vi "Read_Spectro_Variant.vi"(8 "error in (no error)":errorcluster, 9 "Variant":variant, 10 "SpectroCluster":T1) -> (0 "error out":errorcluster, 2 "SpectroCluster":T1)   [LabVIEW 2023, in "Spectrometer Library.lvlib" / "SpectrometerUI.lvlib"]
uses:
  SpectrometerUI.lvlib
  typedefs/SpectroData.ctl
  <userlib>/_OpenG.lib/lvdata/lvdata.llb/openg_variant.lvlib
  typedefs/typedefs.lvlib
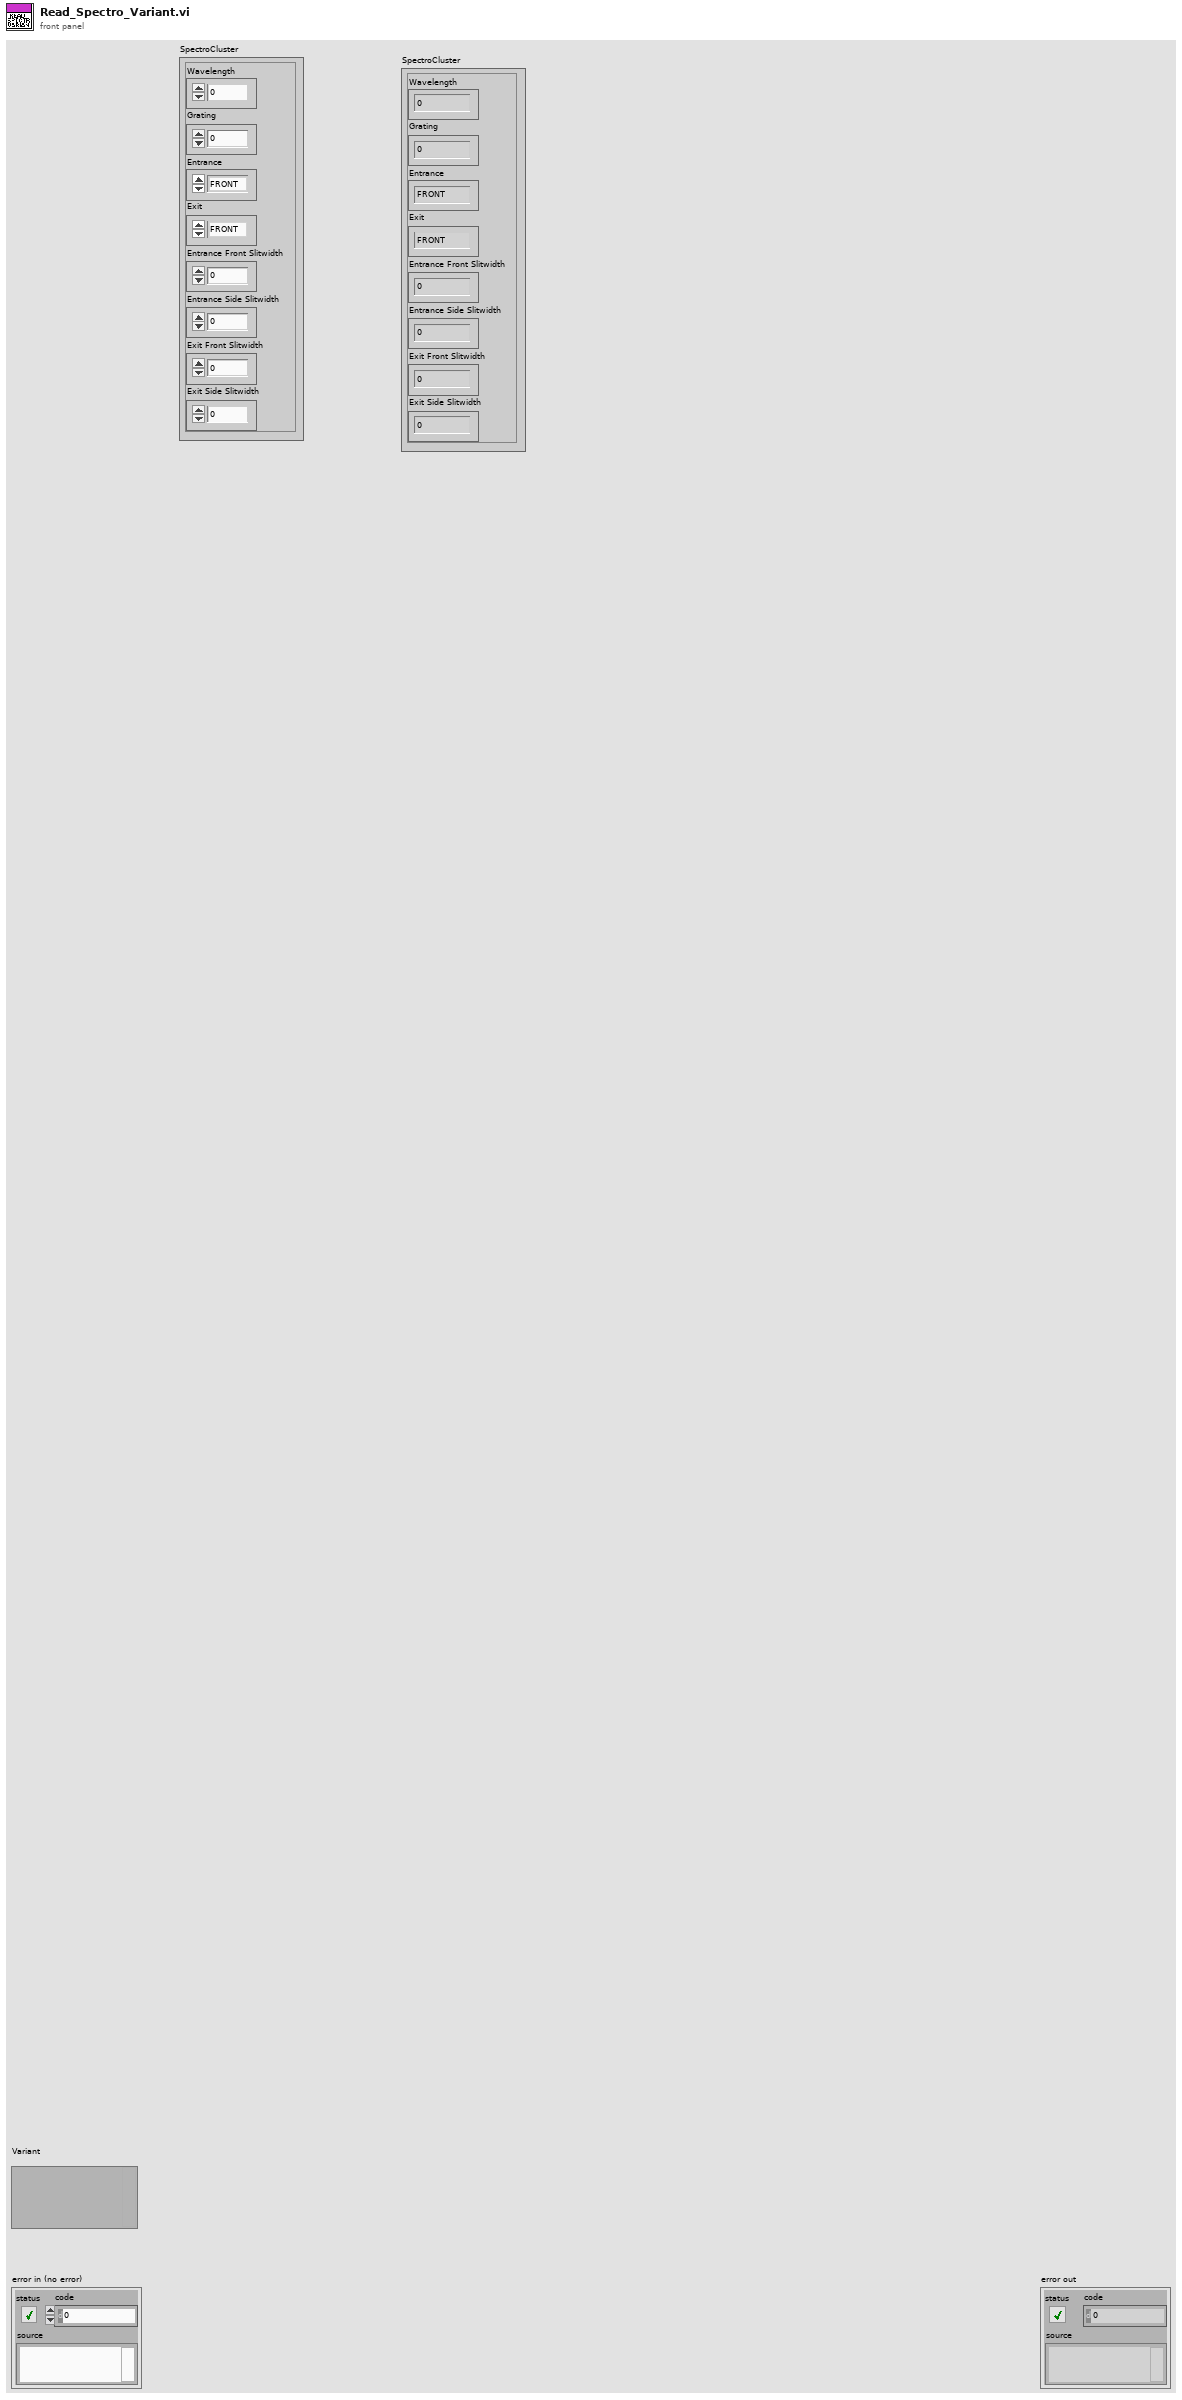
[diagram p1: front panel]
types:
  T1 = typedef "typedefs.lvlib/SpectroData.ctl" = cluster{"Wavelength":dbl, "Grating":u8, "Entrance ":enum16{"FRONT", "SIDE"}, "Exit ":enum16{"FRONT", "SIDE"}, "Entrance Front Slitwidth":u16, "Entrance Side Slitwidth":u16, "Exit Front Slitwidth":u16, "Exit Side Slitwidth":u16}
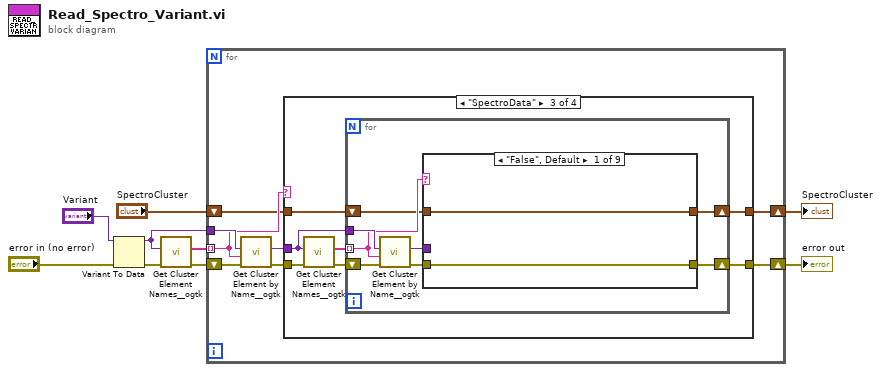
[diagram p0: block diagram]
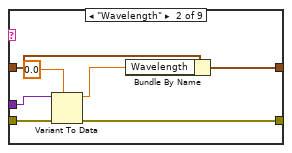
[diagram p4: hidden frame]
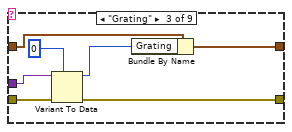
[diagram p5: hidden frame]
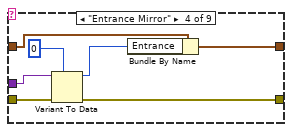
[diagram p6: hidden frame]
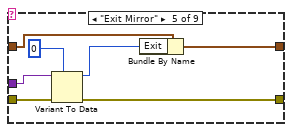
[diagram p7: hidden frame]
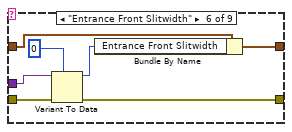
[diagram p8: hidden frame]
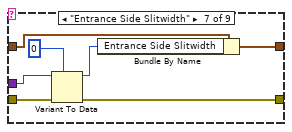
[diagram p9: hidden frame]
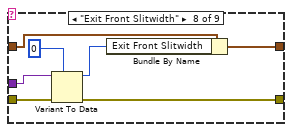
[diagram p10: hidden frame]
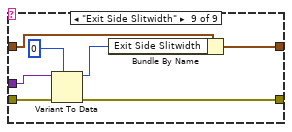
[diagram p11: hidden frame]
diagram:
  n1 = Variant To Data(error in="error in (no error)", Variant="Variant") -> (data=w6:variant, error out=w8:errorcluster)  [unwired: 1 in]
  n2 = call <userlib>:"Get Cluster Element Names__ogtk.vi"("error in (no error)"=w8, "Cluster"=w6) -> ("error out"=w7:errorcluster, "Element Names"=w5:string[])  [unwired: 8 in]
  n3 = for {
    tunnel: w5 -> [w16] mode=indexing
    tunnel: w6 -> [w17]
    shift-right: [w11] -> w9
    shift-left: w7 -> [w12]
    shift-right: [w10] -> w1
    shift-left: "SpectroCluster" -> [w14]
    n4 = call <userlib>:"Get Cluster Element by Name__ogtk.vi"("error in (no error)"=w12, "Element Name"=w16, "Cluster"=w17) -> ("error out"=w13:errorcluster, "VElement"=w15:variant)  [unwired: 6 in, 1 out]
    n5 = case shown="\"SpectroData\"" w16 {
      tunnel: w15 -> [_ _ w27 _]
      tunnel: w14 -> [w19 w21 w26 w96]
      tunnel: [w19 w21 w25 w96] -> w10
      tunnel: w13 -> [w18 w20 w24 w95]
      tunnel: [w18 w20 w22 w95] -> w11
      frame "False", Default {
      }
      frame "InstrError" {
      }
      frame "SpectroData" {
        n6 = call <userlib>:"Get Cluster Element Names__ogtk.vi"("error in (no error)"=w24, "Cluster"=w27) -> ("error out"=w23:errorcluster, "Element Names"=w28:string[])  [unwired: 8 in]
        n7 = for {
          tunnel: w28 -> [w35] mode=indexing
          tunnel: w27 -> [w36]
          shift-right: [w29] -> w22
          shift-left: w23 -> [w31]
          shift-right: [w32] -> w25
          shift-left: w26 -> [w33]
          n8 = call <userlib>:"Get Cluster Element by Name__ogtk.vi"("error in (no error)"=w31, "Element Name"=w35, "Cluster"=w36) -> ("error out"=w30:errorcluster, "VElement"=w34:variant)  [unwired: 6 in, 1 out]
          n9 = case shown="\"False\", Default" w35 {
            tunnel: w34 -> [_ w45 w52 w59 w66 w73 w80 w87 w94]
            tunnel: w33 -> [w38 w42 w50 w56 w64 w71 w78 w85 w92]
            tunnel: [w38 w41 w49 w55 w63 w69 w76 w83 w90] -> w32
            tunnel: w30 -> [w37 w39 w46 w54 w60 w67 w74 w82 w89]
            tunnel: [w37 w40 w47 w53 w61 w68 w75 w81 w88] -> w29
            frame "False", Default {
            }
            frame "Wavelength" {
              n10 = Variant To Data(error in=w39, type=0.0, Variant=w45) -> (data=w43:dbl, error out=w40:errorcluster)
              n11 = Bundle By Name(cluster=w42, "Wavelength"=w43) -> (w41:T1)
            }
            frame "Grating" {
              n12 = Variant To Data(error in=w46, type=u16 0 ("Image XDim"), Variant=w52) -> (data=w48:u16, error out=w47:errorcluster)
              n13 = Bundle By Name(cluster=w50, "Grating"=w48) -> (w49:T1)
            }
            frame "Entrance Mirror" {
              n14 = Variant To Data(error in=w54, type=u16 0 ("Image XDim"), Variant=w59) -> (data=w57:u16, error out=w53:errorcluster)
              n15 = Bundle By Name(cluster=w56, "Entrance"=w57) -> (w55:T1)
            }
            frame "Exit Mirror" {
              n16 = Variant To Data(error in=w60, type=u16 0 ("Image XDim"), Variant=w66) -> (data=w62:u16, error out=w61:errorcluster)
              n17 = Bundle By Name(cluster=w64, "Exit"=w62) -> (w63:T1)
            }
            frame "Entrance Front Slitwidth" {
              n18 = Variant To Data(error in=w67, type=u16 0 ("Image XDim"), Variant=w73) -> (data=w70:u16, error out=w68:errorcluster)
              n19 = Bundle By Name(cluster=w71, "Entrance Front Slitwidth"=w70) -> (w69:T1)
            }
            frame "Entrance Side Slitwidth" {
              n20 = Variant To Data(error in=w74, type=u16 0 ("Image XDim"), Variant=w80) -> (data=w77:u16, error out=w75:errorcluster)
              n21 = Bundle By Name(cluster=w78, "Entrance Side Slitwidth"=w77) -> (w76:T1)
            }
            frame "Exit Front Slitwidth" {
              n22 = Variant To Data(error in=w82, type=u16 0 ("Image XDim"), Variant=w87) -> (data=w84:u16, error out=w81:errorcluster)
              n23 = Bundle By Name(cluster=w85, "Exit Front Slitwidth"=w84) -> (w83:T1)
            }
            frame "Exit Side Slitwidth" {
              n24 = Variant To Data(error in=w89, type=u16 0 ("Image XDim"), Variant=w94) -> (data=w91:u16, error out=w88:errorcluster)
              n25 = Bundle By Name(cluster=w92, "Exit Side Slitwidth"=w91) -> (w90:T1)
            }
          }
        }
      }
      frame "Address" {
      }
    }
  }
  "error out" <- w9
  "SpectroCluster" <- w1
